vi "Variant to Optimizer State.vi"(8 "error in (no error)":errorcluster, 11 "Message Data":variant) -> (0 "error out":errorcluster, 3 "Optimizer State":T1)   [LabVIEW 2020, in "RxnRover.lvlib" / "Generic Optimizer.lvclass"]
doc: "Converts a variant with attributes into a named cluster representing the optimizer state. If a corresponding variant attribute does not exist, the default value for the named element according to the typedef is used."
uses:
  Generic Optimizer.lvclass
  Generic Optimizer State.ctl
  Type Definitions/New Parameters.ctl
  RxnRover.lvlib
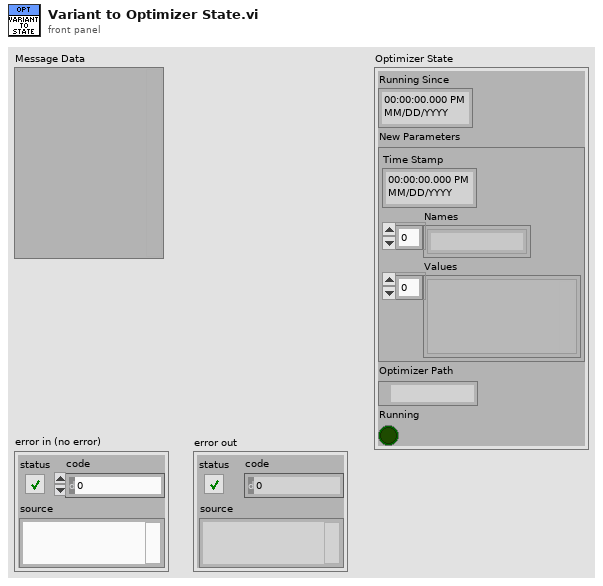
[diagram p1: front panel]
types:
  T1 = typedef "RxnRover.lvlib/Generic Optimizer.lvclass/Generic Optimizer State.ctl" = cluster{"Running Since":timestamp, "New Parameters":T2, "Optimizer Path":path, "Running":bool}
  T2 = typedef "RxnRover.lvlib/New Parameters.ctl" = cluster{"Time Stamp":timestamp, "Names":string[], "Values":variant[]}
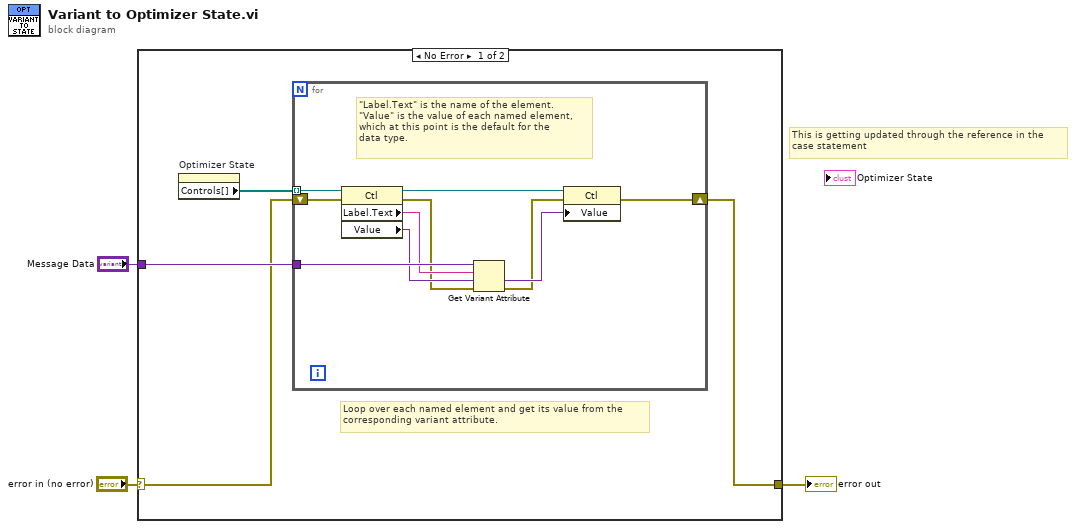
[diagram p0: block diagram]
diagram:
  # "This is getting updated through the reference in the \ncase statement"
  n1 = case shown="No Error" "error in (no error)" {
    selector: "error in (no error)" -> [w5 w18]
    tunnel: [w4 w18] -> w1
    tunnel: "Message Data" -> [w6 _]
    frame No Error {
      # "Loop over each named element and get its value from the\ncorresponding variant attribute."
      n2 = property on="Optimizer State" class="Clust (strict)"() -> ("Controls[]"=w7:refnum<vi>[])  [unwired: 2 in, 2 out]
      n3 = for {
        tunnel: w7 -> [w17] mode=indexing
        tunnel: w6 -> [w16]
        shift-right: [w8] -> w4
        shift-left: w5 -> [w9]
        # "\"Label.Text\" is the name of the element.\n\"Value\" is the value of each named element,\nwhich at this point is the default for the \ndata type."
        n4 = property class="Ctl"(reference=w17, error in=w9) -> (reference out=w13:refnum<vi>, error out=w10:errorcluster, "Label.Text"=w15:string, "Value"=w14:variant)
        n5 = Get Variant Attribute(Variant=w16, name=w15, default value (empty Variant)=w14, error in=w10) -> (value=w12:variant, error out=w11:errorcluster)  [unwired: 2 out]
        n6 = property class="Ctl"(reference=w13, error in=w11, "Value"=w12) -> (error out=w8:errorcluster)  [unwired: 1 out]
      }
    }
    frame Error {
    }
  }
  "error out" <- w1
